vi "AFM_Driver_Manager.ReadActiveDriver.vi"(8 "error in (no error)":errorcluster, 11 "AFM_Driver_Manager in":refnum<class "AFM_Driver_Manager.lvclass">) -> (0 "error out":errorcluster, 2 "Active Driver":T2, 3 "AFM_Driver_Manager out":refnum<class "AFM_Driver_Manager.lvclass">)   [LabVIEW 2019, in "AFM_Driver_Manager.lvclass"]
uses:
  AFM_Driver_Manager.lvclass
  <userlib>/LevyLab/Relay Box/Typedefs/Resistor--enum.ctl
  <userlib>/LevyLab/Relay Box/Relay-Box.lvclass
  AFM_Driver_Manager.PublicMethods.ctl
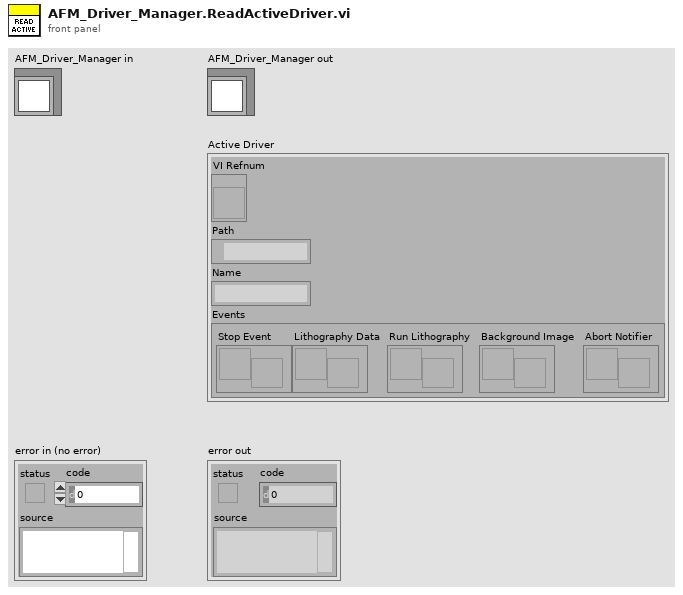
[diagram p1: front panel]
types:
  T1 = typedef "AFM_Driver_Manager.lvclass/AFM_Driver_Manager.PublicMethods.ctl" = cluster{"Stop Event":refnum<user-event>, "Lithography Data":refnum<user-event>, "Run Lithography":refnum<user-event>, "Background Image":refnum<user-event>, "Abort Notifier":refnum<user-event>}
  T2 = cluster{"VI Refnum":refnum<vi>, "Path":path, "Name":string, "Events":T1}
  T3 = cluster{"VI Refnum":refnum<vi>, "Path":path, "Name":string, "Events":T1}[]
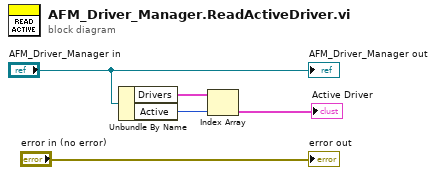
[diagram p0: block diagram]
diagram:
  n1 = Unbundle By Name("AFM_Driver_Manager in") -> ("Drivers"=w2:T3, "Active"=w1:i32)
  n2 = Index Array(array=w2, index=w1) -> (element=→"Active Driver":T2)
  "error out" <- "error in (no error)"
  "AFM_Driver_Manager out" <- "AFM_Driver_Manager in"
